vi "Move Cursor into ROI.vi"(8 "error in (no error)":errorcluster, 11 "Detail Graph in":refnum<class "Detail Graph.lvclass">) -> (0 "error out":errorcluster, 3 "Detail Graph out":refnum<class "Detail Graph.lvclass">)   [LabVIEW 2023, in "Detail Graph.lvclass"]
uses:
  Detail Graph.lvclass
  Detail Graph.lvclass/Detail Graph.ctl
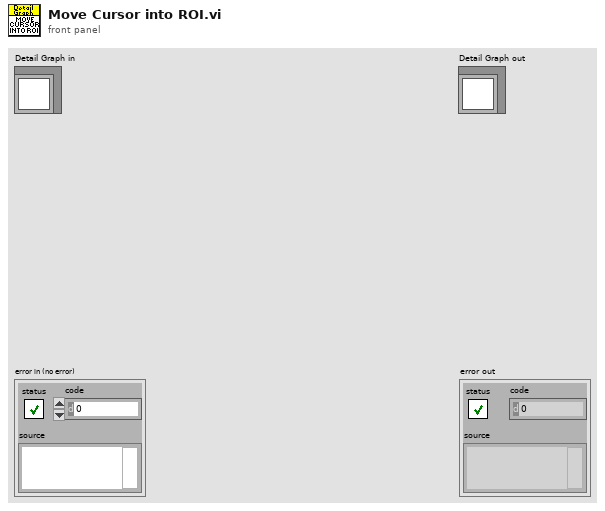
[diagram p1: front panel]
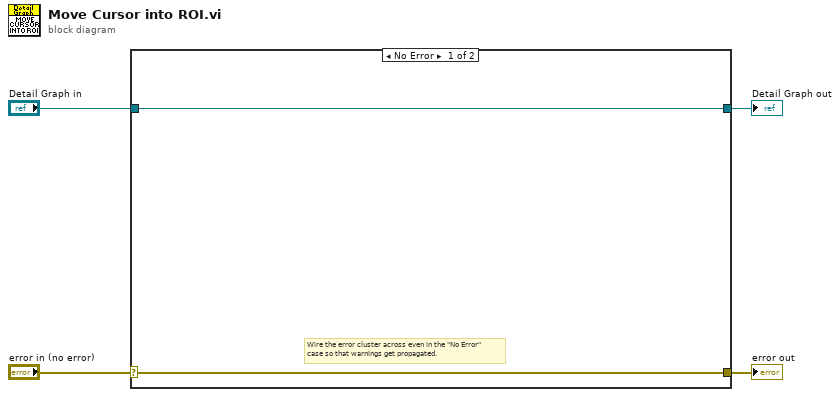
[diagram p0: block diagram]
diagram:
  n1 = case shown="No Error" "error in (no error)" {
    selector: "error in (no error)" -> [w5 w8]
    tunnel: [w5 w8] -> w3
    tunnel: [w6 w7] -> w1
    tunnel: "Detail Graph in" -> [w6 w7]
    frame No Error {
      # "Wire the error cluster across even in the \"No Error\"\ncase so that warnings get propagated."
    }
    frame Error {
    }
  }
  "error out" <- w3
  "Detail Graph out" <- w1
